vi "TOML Example.vi"() -> ()   [LabVIEW 2017]
uses:
  lib/TOML.lvlib
panel:
  out "Parsed Data":T1 {"owner"."dob" format="%<%Y-%m-%d\n%H:%M:%S%3u%z>T"}
  out "TOML String":string
  in  "Tree":string(tree)
  in  "TOML String":string="# This is a TOML document.\n\ntitle = \"TOML Example\"\n\n[owner]\nname = \"David Taylor\"\ndob = 1991-07-17T07:12:00-07:00 # First class dates\n\n[database]\nserver = \"192.168.1.1\"\nports = [ 8001, 8001, 8002 ]\nconnection_max = 5000\nenabled = true\n\n[servers]\n\n  # Indentation (tabs and/or spaces) is allowed but not required\n  [servers.alpha]\n  ip = \"10.0.0.1\"\n  dc = \"eqdc10\"\n\n  [servers.beta]\n  ip = \"10.0.0.2\"\n  dc = \"eqdc10\"\n\n[clients]\ndata = [ [\"gamma\", \"delta\"], [1, 2] ]\n\n# Line breaks are OK when inside arrays\nhosts = [\n  \"alpha\",\n  \"omega\"\n]\n\n#inline table\ninline_table = {one = 1, two = 2}\n\n[[array_of_tables]]\nmulti-line-string = \"\"\"\nline one\nline two\"\"\"\n\n[[array_of_tables]]\nmulti-line-literal-string = '''\nliteral strings allow special characters \\ unescaped\nline two'''"
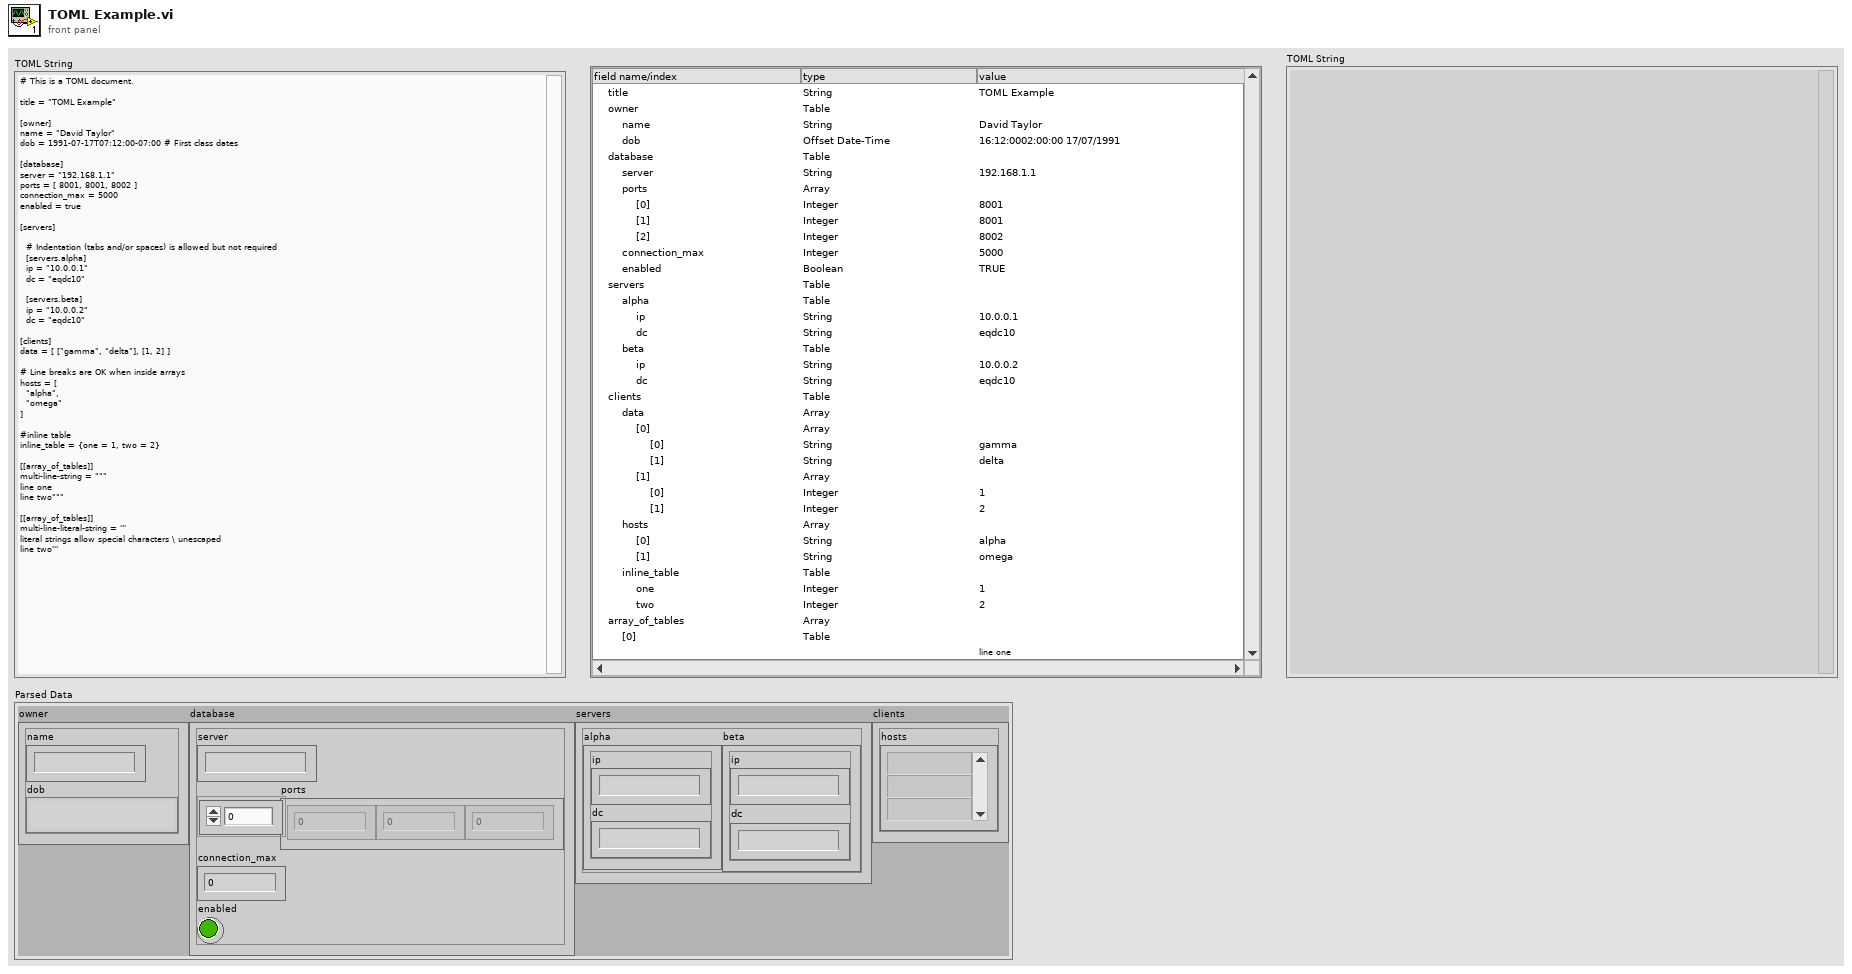
[diagram p1: front panel]
types:
  T1 = cluster{"owner":cluster{"name":string, "dob":timestamp}, "database":cluster{"server":string, "ports":dbl[], "connection_max":dbl, "enabled":bool}, "servers":cluster{"alpha":cluster{"ip":string, "dc":string}, "beta":cluster{"ip":string, "dc":string}}, "clients":cluster{"hosts":string[]}}
  T2 = typedef "TOML.lvlib/TOML Value.ctl" = cluster{"type":enum16{"Table", "Array", "String", "Integer", "Float", "Boolean", "Offset Date-Time", "Local Date-Time", "Local Date", "Local Time"}, "value":variant}
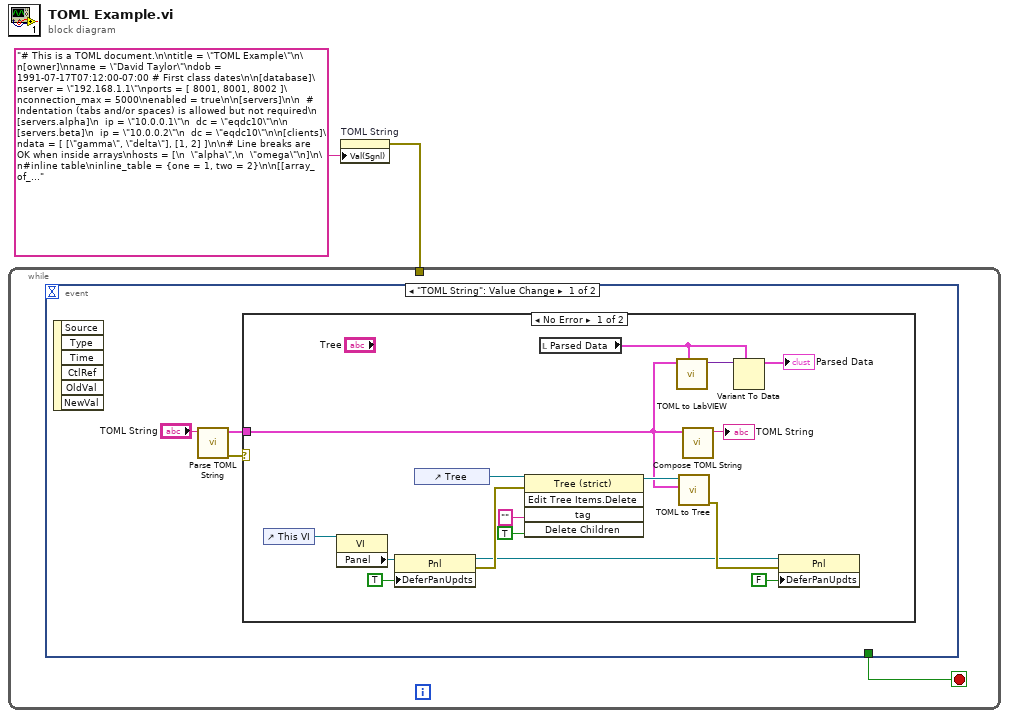
[diagram p0: block diagram]
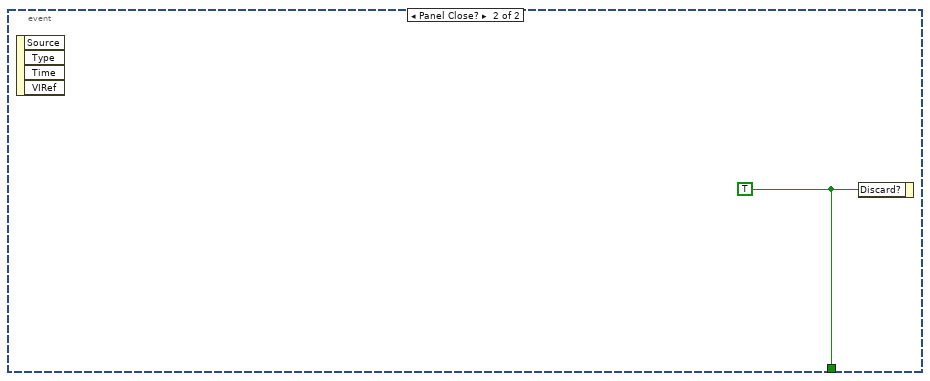
[diagram p3: hidden frame]
diagram:
  n1 = property on="TOML String" class="Str"("Val(Sgnl)"="# This is a TOML document.\n\ntitle = \"TOML Example\"\n\n[owner]\nname = \"David Taylor\"\ndob = 1991-07-17T07:12:00-07:00 # First class dates\n\n[database]\nserver = \"192.168.1.1\"\nports = [ 8001, 8001, 8002 ]\nconnection_max = 5000\nenabled = true\n\n[servers]\n\n  # Indentation (tabs and/or spaces) is allowed but not required\n  [servers.alpha]\n  ip = \"10.0.0.1\"\n  dc = \"eqdc10\"\n\n  [servers.beta]\n  ip = \"10.0.0.2\"\n  dc = \"eqdc10\"\n\n[clients]\ndata = [ [\"gamma\", \"delta\"], [1, 2] ]\n\n# Line breaks are OK when inside arrays\nhosts = [\n  \"alpha\",\n  \"omega\"\n]\n\n#inline table\ninline_table = {one = 1, two = 2}\n\n[[array_of_tables]]\nmulti-line-string = \"\"\"\nline one\nline two\"\"\"\n\n[[array_of_tables]]\nmulti-line-literal-string = '''\nliteral strings allow special characters \\ unescaped\nline two'''" ("TOML String")) -> (error out=w1:errorcluster)  [unwired: 2 in, 1 out]
  n2 = while {
    tunnel: w1 -> [_]
    stop <- w3 stop-if-true
    n3 = event shown="[0] \"TOML String\": Value Change" {
      selector: _ -> [_ _]
      dyn-events: _ -> [_ _]
      timeout: _ -> [_ _]
      tunnel: [_ w23] -> w3
      event "TOML String": Value Change {
        n4 = event-data() -> ()  [unwired: 1 in, 6 out]
        n5 = call "Parse TOML String.vi"("String"="TOML String") -> ("error out"=w6:errorcluster, "Value"=w4:T2)  [unwired: 9 in]
        n6 = case shown="No Error" w6 {
          tunnel: w4 -> [w9 _]
          frame No Error {
            n7 = control-ref of="This VI"() -> (w18:refnum<vi>)
            n8 = property class="VI"(reference=w18) -> ("Panel"=w17:refnum<vi>)  [unwired: 1 in, 2 out]
            n9 = property class="Pnl"(reference=w17, "DeferPanUpdts"=TRUE ("Defer Panel Updates")) -> (reference out=w13:refnum<vi>, error out=w15:errorcluster)  [unwired: 1 in]
            n10 = control-ref of="Tree"() -> (w22:refnum<vi>)
            n11 = invoke class="Tree (strict)" method="Edit Tree Items.Delete"(reference=w22, error in=w15, "tag"="" ("Tag"), "Delete Children"=TRUE ("Delete Children?")) -> (reference out=w19:refnum<vi>)  [unwired: 1 in, 4 out]
            n12 = local read "Parsed Data"() -> (w11:T1)
            n13 = call "TOML to LabVIEW.vi"("Default Value"=w11, "TOML Value"=w9) -> ("LV Value"=w8:variant)  [unwired: 8 in, 1 out]
            n14 = call "TOML to Tree.vi"("Value"=w9, "TreeControl in"=w19) -> ("error out"=w14:errorcluster)  [unwired: 9 in]
            n15 = call "Compose TOML String.vi"("Value"=w9) -> ("String"=→"TOML String":string)  [unwired: 9 in, 1 out]
            n16 = Variant To Data(type=w11, Variant=w8) -> (data=→"Parsed Data":T1)  [unwired: 1 in, 1 out]
            n17 = property class="Pnl"(reference=w13, error in=w14, "DeferPanUpdts"=FALSE ("Defer Panel Updates")) -> ()  [unwired: 2 out]
          }
          frame Error {
          }
        }
      }
      event Panel Close? {
        w23 = TRUE
        n18 = event-data() -> ()  [unwired: 1 in, 4 out]
        n19 = event-data("Discard?"=w23) -> ()  [unwired: 1 in, 1 out]
      }
    }
  }
